vi "Binary to One Hot (U8).vi"(7 "Binary Number":u8 format="%08b") -> (8 "One Hot Encoded Number":u8 format="%08b")   [LabVIEW 2012]
doc: "This code converts Binary U8 to One hot Encoded Number version of leading one detector from MSB.\n\n000011110000 -- input\n111100001111 -- invert\n111100010000 -- add 1\n000000010000 -- and with input.\n\nexample 2:\n1010101011 -- input\n0101010100 -- invert\n0101010101 -- add 1\n0000000001 -- and with input"
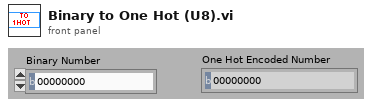
[diagram p1: front panel]
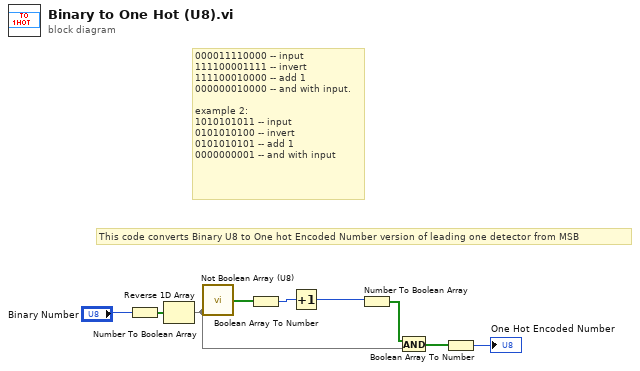
[diagram p0: block diagram]
diagram:
  # "This code converts Binary U8 to One hot Encoded Number version of leading one detector from MSB"
  # "000011110000 -- input\n111100001111 -- invert\n111100010000 -- add 1\n000000010000 -- and with input.\n\nexample 2:\n1010101011 -- input\n0101010100 -- invert\n0101010101 -- add 1\n0000000001 -- and with input"
  n1 = Number To Boolean Array(number="Binary Number") -> (Boolean array=w4:bool[])
  n2 = Reverse 1D Array(array=w4) -> (reversed array=w1:bool[])
  n3 = call <userlib>:"Not Boolean Array (U8).vi"("X"=w1) -> ("Not X"=w9:bool[])  [unwired: 4 in]
  n4 = Boolean Array To Number(Boolean array=w9) -> (number=w8:u8)
  n5 = Increment(x=w8) -> (x+1=w6:u8)
  n6 = Number To Boolean Array(number=w6) -> (Boolean array=w5:bool[])
  n7 = And(x=w5, y=w1) -> (x .and. y?=w3:bool[])
  n8 = Boolean Array To Number(Boolean array=w3) -> (number=→"One Hot Encoded Number":u8)
